vi "Adding Values to an Array by Iterating Through Each Value.vi"(10 "array":dbl[][](array[numeric])) -> (2 "array 2":dbl[][](array[numeric]))   [LabVIEW 2015]
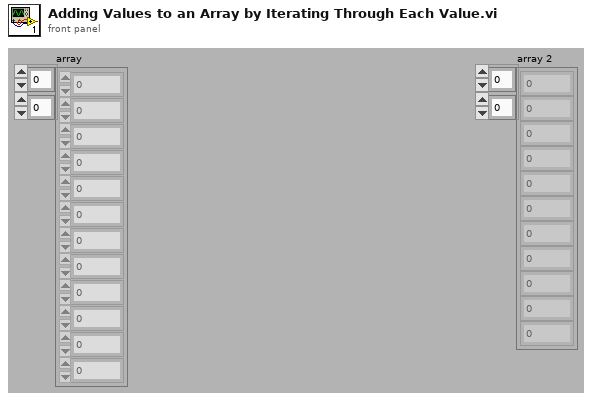
[diagram p1: front panel]
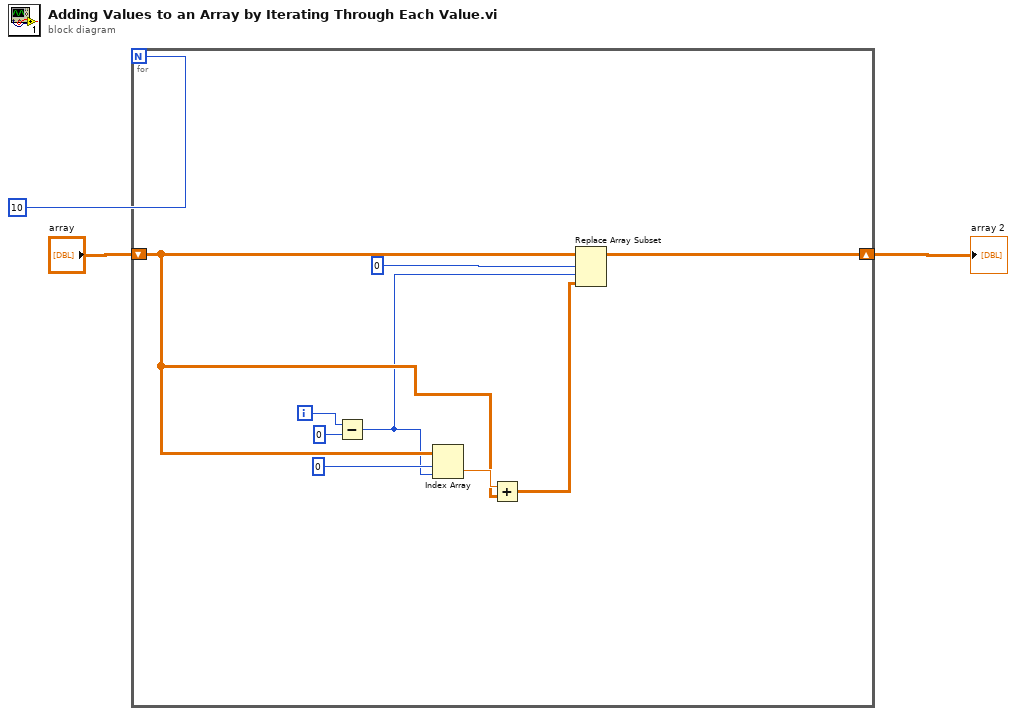
[diagram p0: block diagram]
diagram:
  n1 = for {
    N: 10 -> [_]
    shift-right: [w12] -> w3
    shift-left: "array" -> [w7]
    i -> [w6]
    n2 = Subtract(x=w6, y=0) -> (x-y=w4:i32)
    n3 = Index Array(array=w7, index (row)=0 ("disabled index (row)"), index (col)=w4) -> (element=w9:dbl)
    n4 = Add(x=w9, y=w7) -> (x+y=w8:dbl[][])
    n5 = Replace Array Subset(array=w7, new element=w8, index (row)=0 ("disabled index (row)"), index (col)=w4) -> (w12:dbl[][])
  }
  "array 2" <- w3
